vi "SyncAllReposToLatest.vi"(8 "error in (no error)":errorcluster, 11 "CommandLine":string[](array[string])) -> (0 "error out":errorcluster, 2 "test details":string)   [LabVIEW 2019]
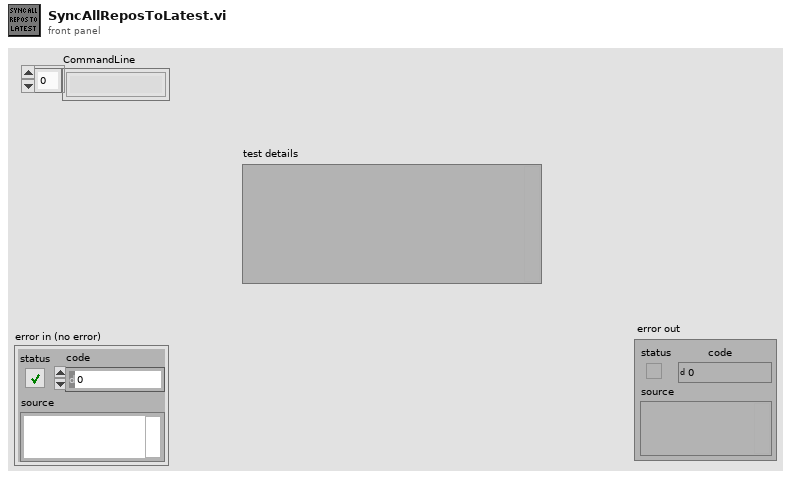
[diagram p1: front panel]
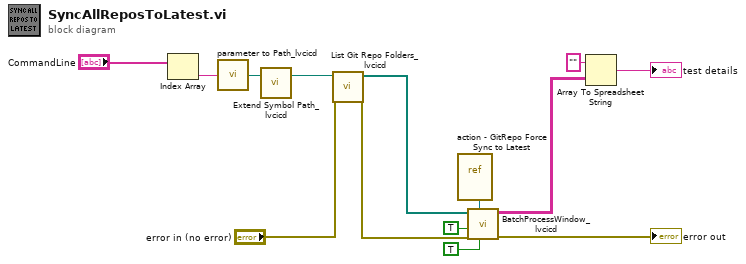
[diagram p0: block diagram]
diagram:
  n1 = Index Array(array="CommandLine") -> (element=w1:string)  [unwired: 1 in]
  n2 = call "parameter to Path_lvcicd.vi"("String"=w1) -> ("Path"=w4:path)
  n3 = call "Extend Symbol Path_lvcicd.vi"("Symbol Path"=w4) -> ("Resolved Path"=w2:path)  [unwired: 2 in]
  n4 = call "List Git Repo Folders_lvcicd.vi"("error in (no error)"="error in (no error)", "path"=w2) -> ("error out"=w10:errorcluster, "Repo Folders"=w13:path[])  [unwired: 8 in]
  n5 = vi-ref "action - GitRepo Force Sync to Latest.vi"() -> (w9:refnum<vi>)
  n6 = call "BatchProcessWindow_lvcicd.vi"("FP(T)"=TRUE, "VI Refnum"=w9, "error in (no error)"=w10, "silence mode(F)"=TRUE, "paths"=w13) -> ("error out"=→"error out":errorcluster, "Array"=w12:string[][])  [unwired: 5 in]
  n7 = Array To Spreadsheet String(array=w12, 3:"" ("format string")) -> (spreadsheet string=→"test details":string)  [unwired: 1 in]
